vi "Turn Angle Calculation with Gyro.vi"(7 "Force Degrees":bool, 8 "Turn Direction":string(combo), 9 "GyroHeading":dbl, 11 "Angle Input":dbl) -> (3 "Angle  Output":dbl)   [LabVIEW 2017]
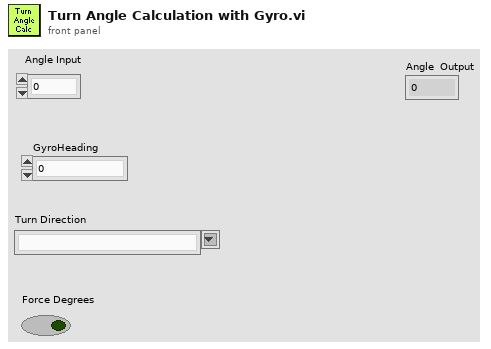
[diagram p1: front panel]
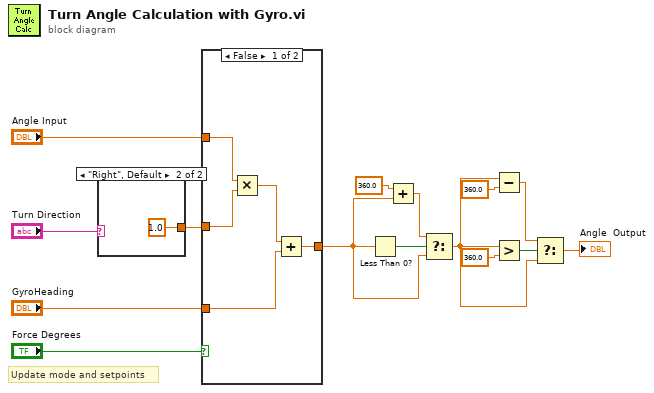
[diagram p0: block diagram]
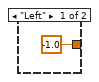
[diagram p2: hidden frame]
diagram:
  # "Update mode and setpoints"
  n1 = case shown="\"Right\", Default" "Turn Direction" {
    tunnel: [-1.0 1.0] -> w13
    frame "Left" {
    }
    frame "Right", Default {
    }
  }
  n2 = case shown="False" "Force Degrees" {
    tunnel: "Angle Input" -> [w22 w23]
    tunnel: [w18 w23] -> w11
    tunnel: "GyroHeading" -> [w19 _]
    tunnel: w13 -> [w21 _]
    frame False {
      n3 = Multiply(x=w22, y=w21) -> (x*y=w20:dbl)
      n4 = Add(x=w20, y=w19) -> (x+y=w18:dbl)
    }
    frame True {
    }
  }
  n5 = Less Than 0?(x=w11) -> (x < 0?=w12:bool)
  n6 = Add(x=360.0, y=w11) -> (x+y=w9:dbl)
  n7 = Select(t=w9, s=w12, f=w11) -> (s? t:f=w6:dbl)
  n8 = Subtract(x=w6, y=360.0) -> (x-y=w4:dbl)
  n9 = Greater?(x=w6, y=360.0) -> (0:w7:bool)
  n10 = Select(t=w4, s=w7, f=w6) -> (s? t:f=→"Angle  Output":dbl)
